vi "Double_Card_Config.vi"(2 "错误输入":errorcluster caption="错误输入（无错误）", 3 "单通道采样率(Hz)":i32=1000) -> (0 "错误输出":errorcluster, 1 "DevOut":i32)   [LabVIEW 2018]
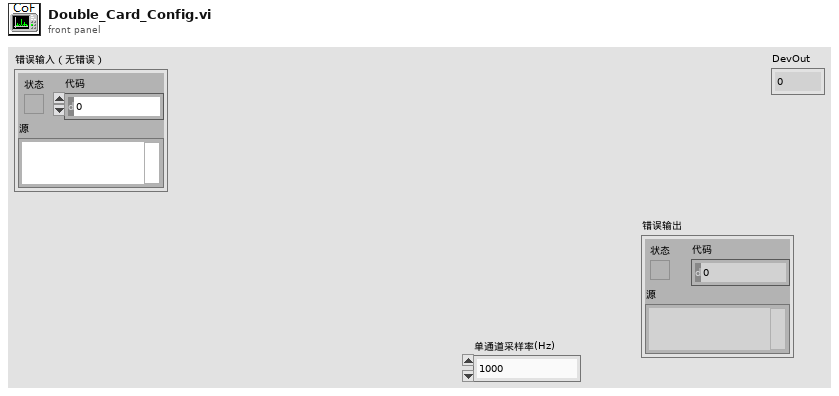
[diagram p1: front panel]
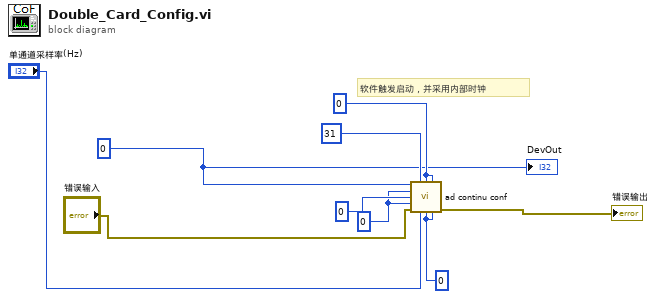
[diagram p0: block diagram]
diagram:
  w2 = 0 ("dev")
  w4 = 0 ("trig_pol")
  w6 = 0 ("trig_sl")
  w8 = 0 ("ch_first")
  # "软件触发启动，并采用内部时钟"
  n1 = call "ad continu conf.vi"("dev"=w2, "ch_last"=31, "trig_sl"=w6, "clk_sl"=w6, "ad_os"=w8, "ad_range"=0, "ch_first"=w8, "error in (no error)"="错误输入", "freq"="单通道采样率(Hz)", "trig_pol"=w4, "ext_clk_pol"=w4) -> ("error out"=→"错误输出":errorcluster)  [unwired: 3 in, 1 out]
  "DevOut" <- w2
